vi "Process.vi"(8 "error in (no error)":errorcluster, 10 "pound in":refnum<class "Pound.lvclass">, 11 "qbus in":refnum<class "Qbus.lvclass">) -> (0 "error out":errorcluster)   [LabVIEW 2015, in "DeleteProcess.lvlib"]
doc: "Implements timer tasks that other processes register by sending Qbus messages to those processes."
uses:
  DeleteProcess.lvlib
  <vilib>/addons/Qbus/Qbus.lvclass
  <vilib>/NI/Software Watchdog/Pound/Pound.lvclass
  controls/ProcessState.ctl
  FileHandler/controls/FileForDelete.ctl
  <vilib>/NI/Software Watchdog/Watchdog/Watchdog.lvclass
  FileHandler/FileHandler.lvlib
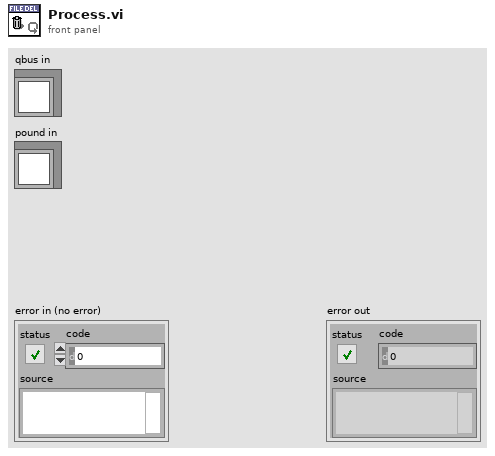
[diagram p1: front panel]
types:
  T1 = typedef "DeleteProcess.lvlib/ProcessState.ctl" = cluster{"FileForDelete":T2}
  T2 = typedef "FileHandler.lvlib/FileForDelete.ctl" = cluster{"Last File Time":timestamp, "Paths":path[]}
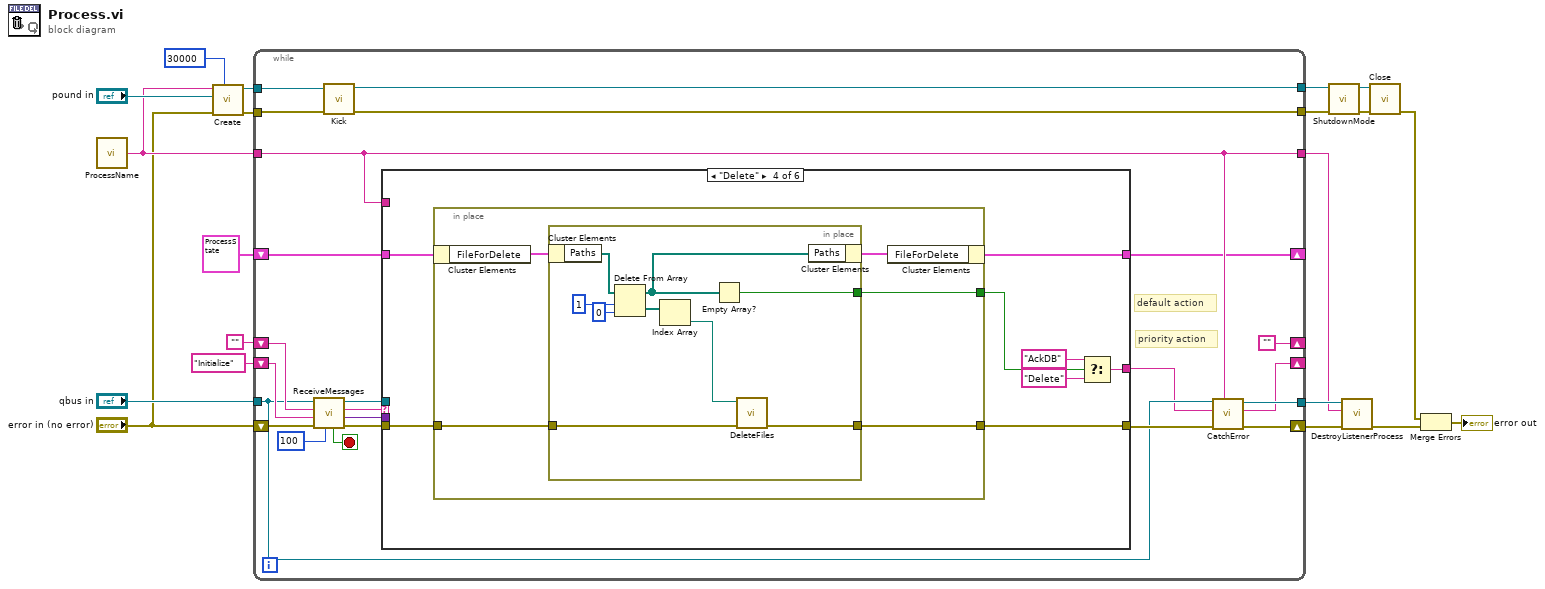
[diagram p0: block diagram]
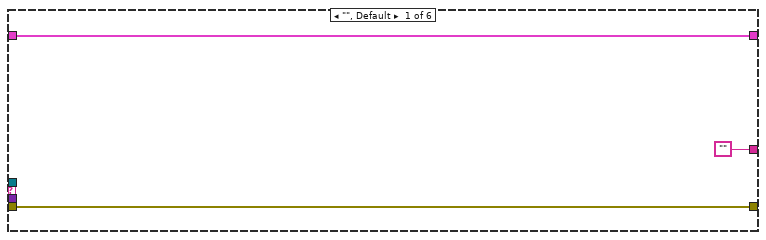
[diagram p2: hidden frame]
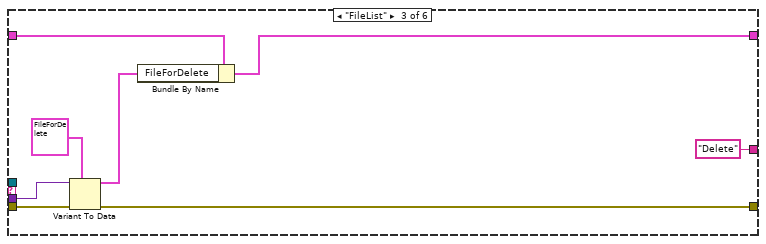
[diagram p4: hidden frame]
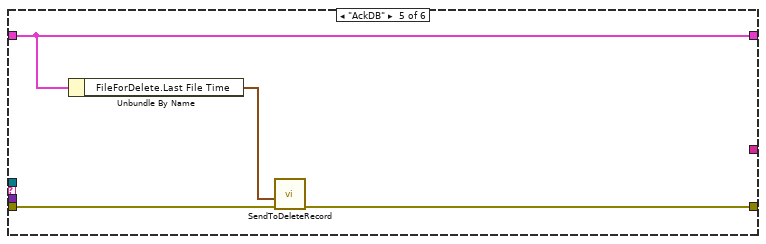
[diagram p5: hidden frame]
diagram:
  n1 = call "ProcessName.vi"() -> ("process name"=w11:string)  [unwired: 5 in]
  n2 = call <vilib>:"Create.vi"("Execution Timeout (ms)"=u32 30000, "error in (no error)"="error in (no error)", "Pound"="pound in", "Name"=w11) -> ("error out"=w13:errorcluster, "Watchdog"=w12:refnum<data-value>)  [unwired: 6 in]
  n3 = while {
    shift-right: [""] -> _
    shift-left: "" -> [w41]
    tunnel: "qbus in" -> [w25]
    tunnel: w11 -> [w32]
    tunnel: [w34] -> w18
    tunnel: [w32] -> w17
    shift-right: [w33] -> _
    shift-left: "Initialize" -> [w36]
    tunnel: w13 -> [w30]
    tunnel: w12 -> [w29]
    tunnel: [w28] -> w6
    tunnel: [w27] -> w7
    shift-right: [w35] -> w19
    shift-left: "error in (no error)" -> [w43]
    shift-right: [w22] -> _
    shift-left: T1 {"FileForDelete"={"Last File Time"=timestamp(0 s since 1904-01-01), "Paths"=[]}} ("ProcessState") -> [w23]
    stop <- w42 stop-if-true
    # "priority action"
    # "default action"
    n4 = call "ReceiveMessages.vi"("timeout(100)"=100, "error in (no error)"=w43, "priority action"=w36, "default action"=w41, "qbus in"=w25) -> ("error out"=w40:errorcluster, "message value"=w37:variant, "action"=w26:string, "qbus out"=w38:refnum<class "Qbus.lvclass">, "exit"=w42:bool)  [unwired: 2 in]
    n5 = call <vilib>:"Kick.vi"("error in (no error)"=w30, "Watchdog"=w29) -> ("error out"=w27:errorcluster, "Watchdog"=w28:refnum<data-value>)  [unwired: 8 in]
    n6 = case shown="\"Delete\"" w26 {
      tunnel: w40 -> [w46 w47 w56 w63 w81 w83]
      tunnel: w38 -> [_ _ _ _ _ _]
      tunnel: [w46 w47 w53 w61 w79 w83] -> w31
      tunnel: w37 -> [_ _ w55 _ _ _]
      tunnel: w32 -> [_ _ _ _ _ _]
      tunnel: w23 -> [w45 w48 w52 w64 w82 w84]
      tunnel: [w45 w48 w50 w62 w82 w84] -> w22
      tunnel: ["" _ "Delete" w58 _ _] -> w21
      frame "", Default {
      }
      frame "Initialize" {
      }
      frame "FileList" {
        n7 = Variant To Data(error in=w56, type=T2 {"Last File Time"=timestamp(0 s since 1904-01-01), "Paths"=[]} ("FileForDelete"), Variant=w55) -> (data=w51:T2, error out=w53:errorcluster)
        n8 = Bundle By Name(cluster=w52, "FileForDelete"=w51) -> (w50:T1)
      }
      frame "Delete" {
        n9 = in-place {
          in-place-border: w63 -> [w67]
          in-place-border: [w66] -> w61
          in-place-border: [w65] -> w60
          n10 = in-place-cluster #1(w64) -> ("FileForDelete"=w69:T2)
          n11 = in-place {
            in-place-border: w67 -> [w71]
            in-place-border: [w72] -> w66
            in-place-border: [w73] -> w65
            n12 = in-place-cluster #2(w69) -> ("Paths"=w78:path[])
            n13 = Delete From Array(array=w78, length=1, index=0) -> (deleted portion=w75:path[], array with subset deleted=w74:path[])
            n14 = Index Array(array=w75) -> (element=w70:path)  [unwired: 1 in]
            n15 = Empty Array?(array=w74) -> (empty?=w73:bool)
            n16 = call "DeleteFiles.vi"("error in (no error)"=w71, "Path"=w70) -> ("error out"=w72:errorcluster)  [unwired: 9 in]
            n17 = in-place-cluster #2("Paths"=w74) -> (w68:T2)
          }
          n18 = in-place-cluster #1("FileForDelete"=w68) -> (w62:T1)
        }
        n19 = Select(t="AckDB", s=w60, f="Delete") -> (s? t:f=w58:string)
      }
      frame "AckDB" {
        n20 = Unbundle By Name(w82) -> ("FileForDelete.Last File Time"=w80:timestamp)
        n21 = call "SendToDeleteRecord.vi"("error in (no error)"=w81, "message value"=w80) -> ("error out"=w79:errorcluster)  [unwired: 9 in]
      }
      frame "Exit" {
      }
    }
    n22 = call <vilib>:"CatchError.vi"("source"=w32, "error in (no error)"=w31, "next action in"=w21, "Qbus in"=w25) -> ("error out"=w35:errorcluster, "next action out"=w33:string, "Qbus out"=w34:refnum<class "Qbus.lvclass">)  [unwired: 5 in]
  }
  n23 = call <vilib>:"ShutdownMode.vi"("error in (no error)"=w7, "Watchdog"=w6) -> ("error out"=w8:errorcluster, "Watchdog"=w9:refnum<data-value>)  [unwired: 8 in]
  n24 = call <vilib>:"DestroyListenerProcess.vi"("error in (no error)"=w19, "process name"=w17, "Qbus in"=w18) -> ("error in (no error)"=w4:errorcluster)  [unwired: 7 in, 1 out]
  n25 = call <vilib>:"Close.vi"("error in (no error)"=w8, "Watchdog"=w9) -> ("error out"=w5:errorcluster)  [unwired: 9 in]
  n26 = Merge Errors(w5, w4) -> (→"error out":errorcluster)
